vi "Update Scan Table.vi"(7 "Scan Table Ref":refnum<vi>, 8 "error in (no error)":errorcluster, 11 "Scanned Addresses Ref":refnum<vi>) -> (0 "error out":errorcluster)   [LabVIEW 2025, in "I2C Bus Monitor UI.lvlib"]
uses:
  I2C Bus Monitor UI.lvlib
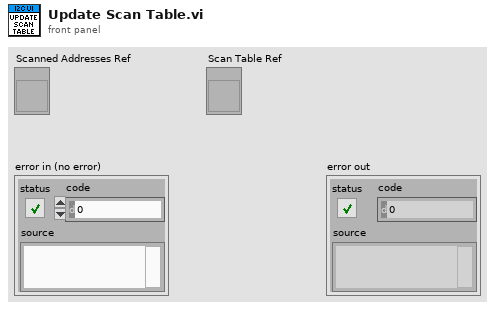
[diagram p1: front panel]
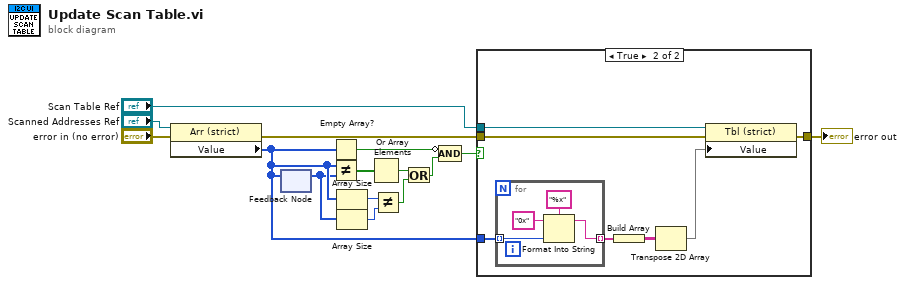
[diagram p0: block diagram]
diagram:
  n1 = property class="Arr (strict)"(reference="Scanned Addresses Ref", error in="error in (no error)") -> (error out=w13:errorcluster, "Value"=w5:i32[])  [unwired: 1 out]
  n2 = feedback #1() -> (w4:i32[])  [unwired: 1 in]
  n3 = feedback-in #1(w5) -> ()
  n4 = Empty Array?(array=w5) -> (empty?=w9:bool)
  n5 = Not Equal?(x=w5, y=w4) -> (x != y?=w10:bool[])
  n6 = Array Size(array=w5) -> (size(s)=w3:i32)
  n7 = Array Size(array=w4) -> (size(s)=w2:i32)
  n8 = Or Array Elements(Boolean array=w10) -> (logical OR=w7:bool)
  n9 = Not Equal?(x=w3, y=w2) -> (x != y?=w1:bool)
  n10 = Or(x=w7, y=w1) -> (x .or. y?=w6:bool)
  n11 = Compound Arithmetic op=AND(invert w9, w6) -> (w8:bool)
  n12 = case shown="True" w8 {
    tunnel: [w16 w23] -> w14
    tunnel: w13 -> [w16 w22]
    tunnel: w5 -> [_ w21]
    tunnel: "Scan Table Ref" -> [_ w20]
    frame False {
    }
    frame True {
      n13 = for {
        tunnel: w21 -> [w25] mode=indexing
        tunnel: [w24] -> w18 mode=indexing
        n14 = Format Into String(format string="%x", initial string="0x", w25) -> (resulting string=w24:string)  [unwired: 1 in, 1 out]
      }
      n15 = Build Array(w18) -> (w19:string[][])
      n16 = Transpose 2D Array(2D array=w19) -> (transposed array=w17:string[][])
      n17 = property class="Tbl (strict)"(reference=w20, error in=w22, "Value"=w17) -> (error out=w23:errorcluster)  [unwired: 1 out]
    }
  }
  "error out" <- w14
